vi "transform cluster data to XY graph.vi"(11 "data cluster array":cluster{"Slide":dbl, u32[]}[](array[cluster])) -> (3 "XY data":cluster{dbl[], dbl[]}[](array[cluster]))   [LabVIEW 2012]
uses:
  <vilib>/vision/NI_Vision_Development_Module.lvlib
  <vilib>/Analysis/NI_AALBase.lvlib
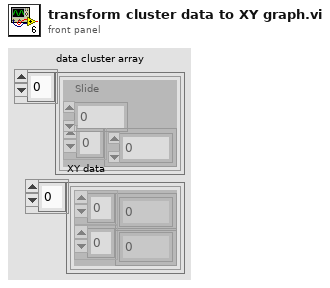
[diagram p1: front panel]
types:
  T1 = cluster{"Red (or Hue) value":u8, "Green (or Sat) value":u8, "Blue (or Light or Val) value":u8}
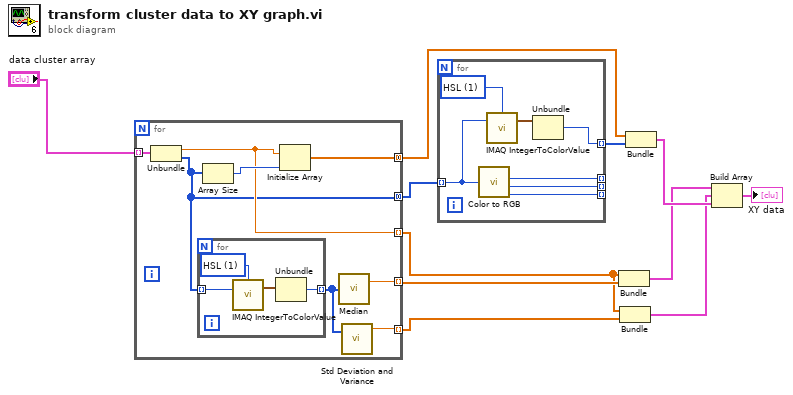
[diagram p0: block diagram]
diagram:
  n1 = for {
    tunnel: "data cluster array" -> [w18] mode=indexing
    tunnel: [w17] -> w11 mode=concatenating
    tunnel: [w15] -> w9 mode=concatenating
    tunnel: [w16] -> w6 mode=indexing
    tunnel: [w14] -> w8 mode=indexing
    tunnel: [w12] -> w7 mode=indexing
    n2 = Unbundle(w18) -> ("Slide"=w16:dbl, w15:u32[])
    n3 = for {
      tunnel: w15 -> [w23] mode=indexing
      tunnel: [w20] -> w13 mode=indexing
      w21 = u16 1 items=["RGB", "HSL", "HSV", "HSI"] ("Color Mode")
      n4 = call "IMAQ IntegerToColorValue"("U32 value"=w23, "Color Mode"=w21) -> ("Color Value"=w22:T1)  [unwired: 3 in, 3 out]
      n5 = Unbundle(w22) -> ("Green (or Sat) value"=w20:u8)  [unwired: 2 out]
    }
    n6 = Array Size(array=w15) -> (size(s)=w19:i32)
    n7 = Initialize Array(w16, w19) -> (w17:dbl[])
    n8 = call <vilib>:"Median.vi"("X"=w13) -> ("median"=w14:dbl)  [unwired: 1 out]
    n9 = call <vilib>:"Std Deviation and Variance.vi"("X"=w13) -> ("mean"=w12:dbl)  [unwired: 1 in, 2 out]
  }
  n10 = for {
    tunnel: w9 -> [w26] mode=indexing
    tunnel: [w30] -> _ mode=indexing
    tunnel: [w29] -> _ mode=indexing
    tunnel: [w28] -> _ mode=indexing
    tunnel: [w24] -> w10 mode=indexing
    w27 = u16 1 items=["RGB", "HSL", "HSV", "HSI"] ("Color Mode")
    n11 = call <vilib>:"Color to RGB.vi"("Color"=w26) -> ("R"=w30:u8, "G"=w29:u8, "B"=w28:u8)  [unwired: 1 out]
    n12 = call "IMAQ IntegerToColorValue"("U32 value"=w26, "Color Mode"=w27) -> ("Color Value"=w25:T1)  [unwired: 3 in, 3 out]
    n13 = Unbundle(w25) -> ("Green (or Sat) value"=w24:u8)  [unwired: 2 out]
  }
  n14 = Bundle(w6, w8) -> (w3:cluster{dbl[], dbl[]})  [unwired: 1 in]
  n15 = Bundle(w6, w7) -> (w4:cluster{dbl[], dbl[]})  [unwired: 1 in]
  n16 = Bundle(w11, w10) -> (w5:cluster{dbl[], u8[]})  [unwired: 1 in]
  n17 = Build Array(w3, w4, w5) -> (→"XY data":cluster{dbl[], dbl[]}[])
